vi "Close.vi"(8 "Error In":errorcluster, 11 "reference in":refnum<class "Thermometer Multichannel.lvclass">) -> (0 "Error Out":errorcluster, 3 "reference out":refnum<class "Thermometer Multichannel.lvclass">)   [LabVIEW 2024, in "Thermometer Multichannel.lvclass"]
uses:
  Thermometer Multichannel.lvclass
  Thermometer Multichannel.lvclass/Thermometer Multichannel.ctl
  Interfaces/IConfigure/IConfigure.lvclass
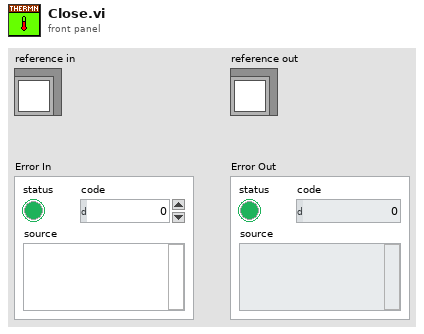
[diagram p1: front panel]
types:
  T1 = typedef "Thermometer Multichannel.lvclass/ObjectAttributes.ctl" = cluster{"IConfigure":refnum<class "IConfigure.lvclass">, "Worker Enqueuer":refnum<class "Message Enqueuer.lvclass">}
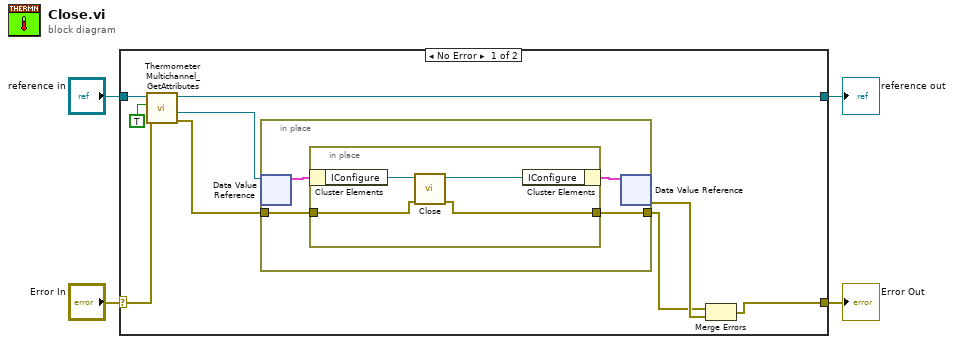
[diagram p0: block diagram]
diagram:
  n1 = case shown="No Error" "Error In" {
    selector: "Error In" -> [w13 w23]
    tunnel: [w5 w23] -> w3
    tunnel: [w11 w22] -> w1
    tunnel: "reference in" -> [w12 w22]
    frame No Error {
      n2 = call "Thermometer Multichannel_GetAttributes.vi"("Error In"=w13, "OnlyGetDvrReference(False)"=TRUE, "reference in"=w12) -> ("Error Out"=w7:errorcluster, "DataRef"=w8:refnum<data-value>, "reference out"=w11:refnum<class "Thermometer Multichannel.lvclass">)  [unwired: 5 in, 1 out]
      n3 = in-place {
        in-place-border: w7 -> [w15]
        in-place-border: [w14] -> w6
        n4 = in-place-dvr #1(w8) -> (w17:T1)  [unwired: 1 out]
        n5 = in-place {
          in-place-border: w15 -> [w19]
          in-place-border: [w18] -> w14
          n6 = in-place-cluster #2(w17) -> ("IConfigure"=w21:refnum<class "IConfigure.lvclass">)
          n7 = call-dynamic "Close.vi"("error in"=w19, "IClose in"=w21) -> ("error out"=w18:errorcluster, "IClose out"=w20:refnum<class "IConfigure.lvclass">)  [unwired: 8 in]
          n8 = in-place-cluster #2("IConfigure"=w20) -> (w16:T1)
        }
        n9 = in-place-dvr #1(w16) -> (w9:errorcluster)  [unwired: 1 out]
      }
      n10 = Merge Errors(w6, w9) -> (w5:errorcluster)
    }
    frame Error {
    }
  }
  "Error Out" <- w3
  "reference out" <- w1
